vi "设备-初始化配置.vi"() -> ()   [LabVIEW 2013]
uses:
  <vilib>/Instr/_visa.llb/VISA Configure Serial Port (Instr).vi
panel:
  out "配置服务器VI引用":refnum<vi>
  out "账户信息":string caption="* 提示："
  out "服务器？":bool
  out "路由？":bool
  out "通信？":bool
  in  "刷新服务器":bool
  in  "连接的设备":i32(listbox)
  in  "配置开关":bool
  out "配置进度":dbl(slide) scale=0.0..1.0
  out "本机IP":string
  out "IP":string
  out "端口":u16
  in  "当前配置流程":T1(ring)
  in  "连续配置":bool=TRUE
  out "MAC":string
  out "查MAC回复":string
  in  "路由密码":string caption="* 路由密码"
  out "路由名称":string
  in  "通信接口":refnum<visa-resource-name> caption="* 通信接口"
  # "已连接设备"
  # "与设备连接"
  # "设备连接到路由器"
  # "设备连接到服务器"
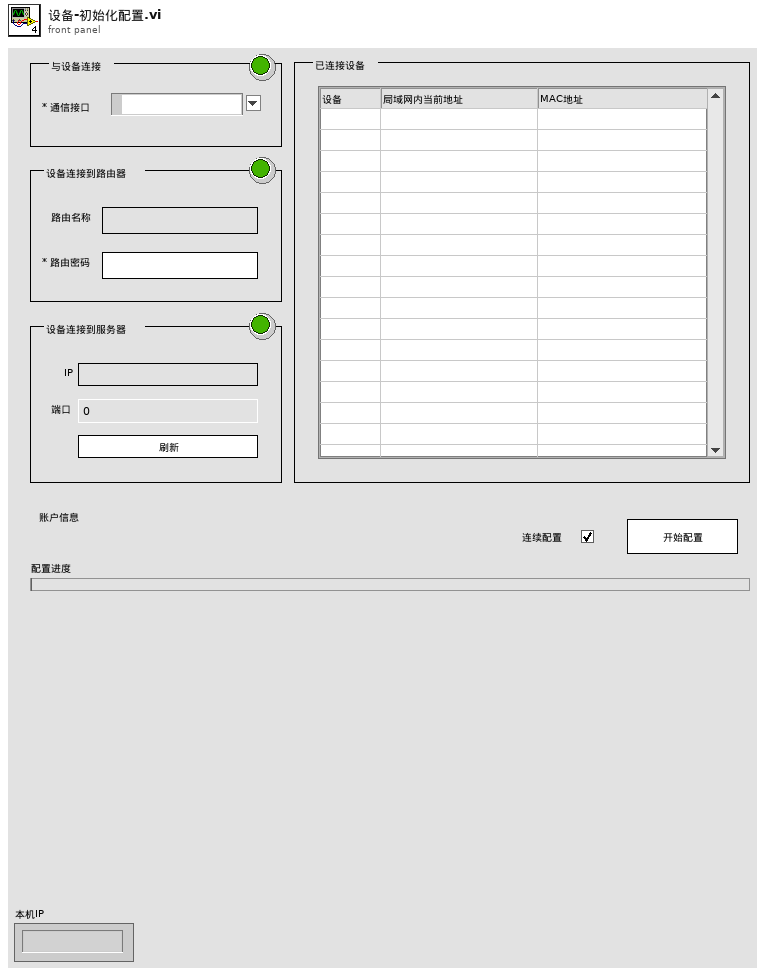
[diagram p1: front panel]
types:
  T1 = enum16{"退出透传", "进入AT指令", "退出AP连接", "设为STA", "连接指定AP", "设为STA开机自连", "获取MAC地址", "禁用智能连接", "透传接收", "连接至配置服务器", "进入透传发送", "等待云服务器端确认", "配置完成"}
  T2 = enum8{"Enabled", "Disabled", "Disabled and Grayed Out"}
  T3 = cluster{"服务器信息":cluster{"IP":string, "Port":u16}, "账户信息":cluster{"账户可用？":bool, "用户名":string, "密码":string}}
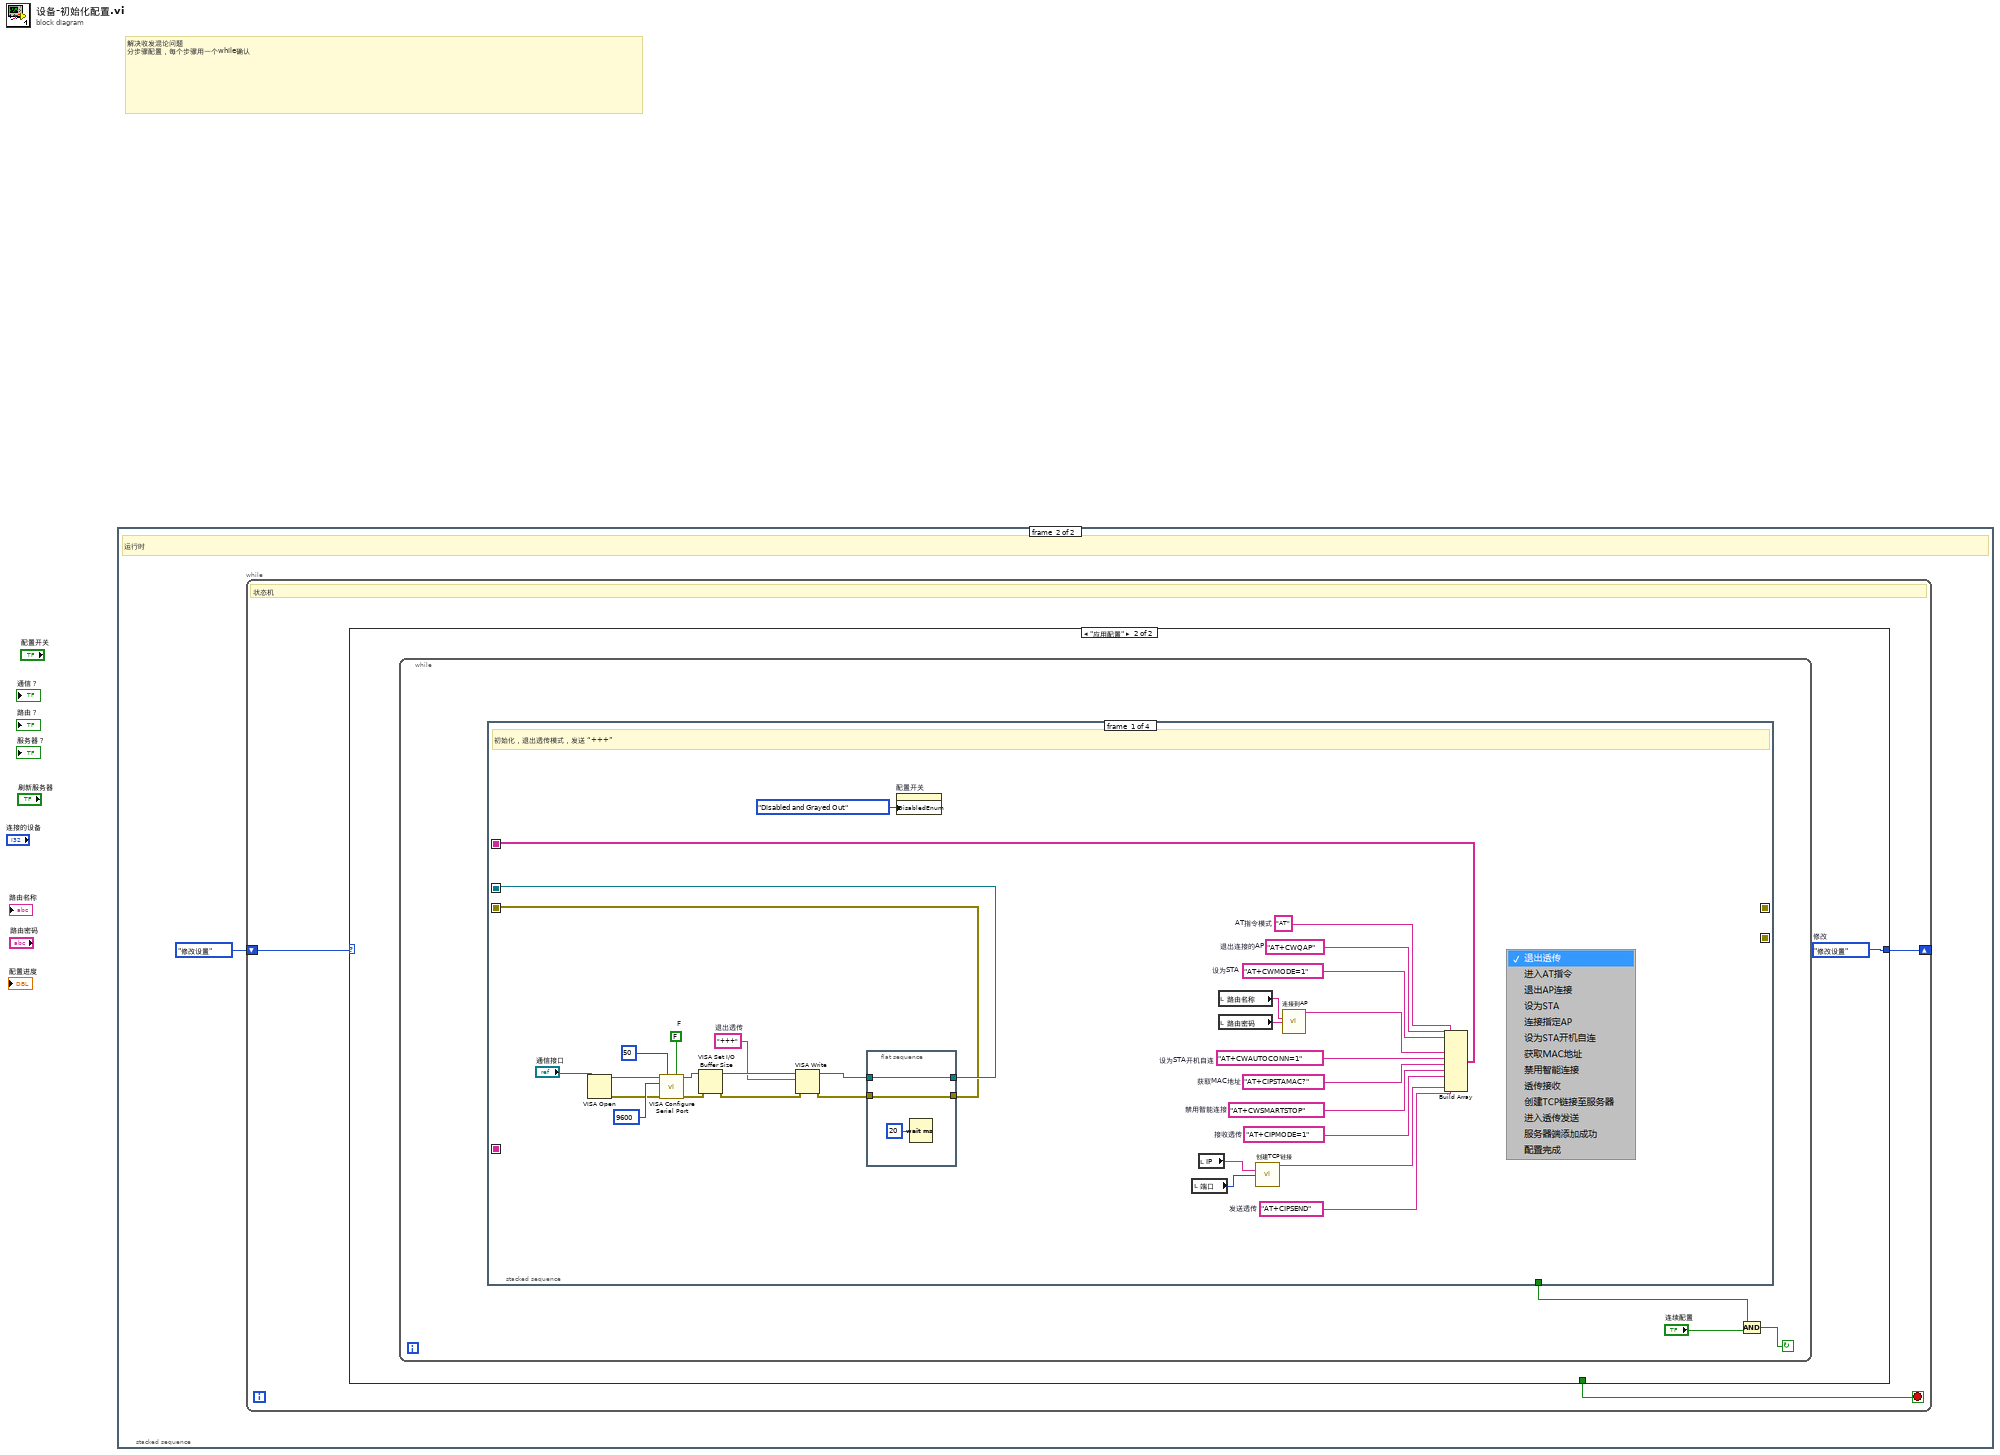
[diagram p0: block diagram]
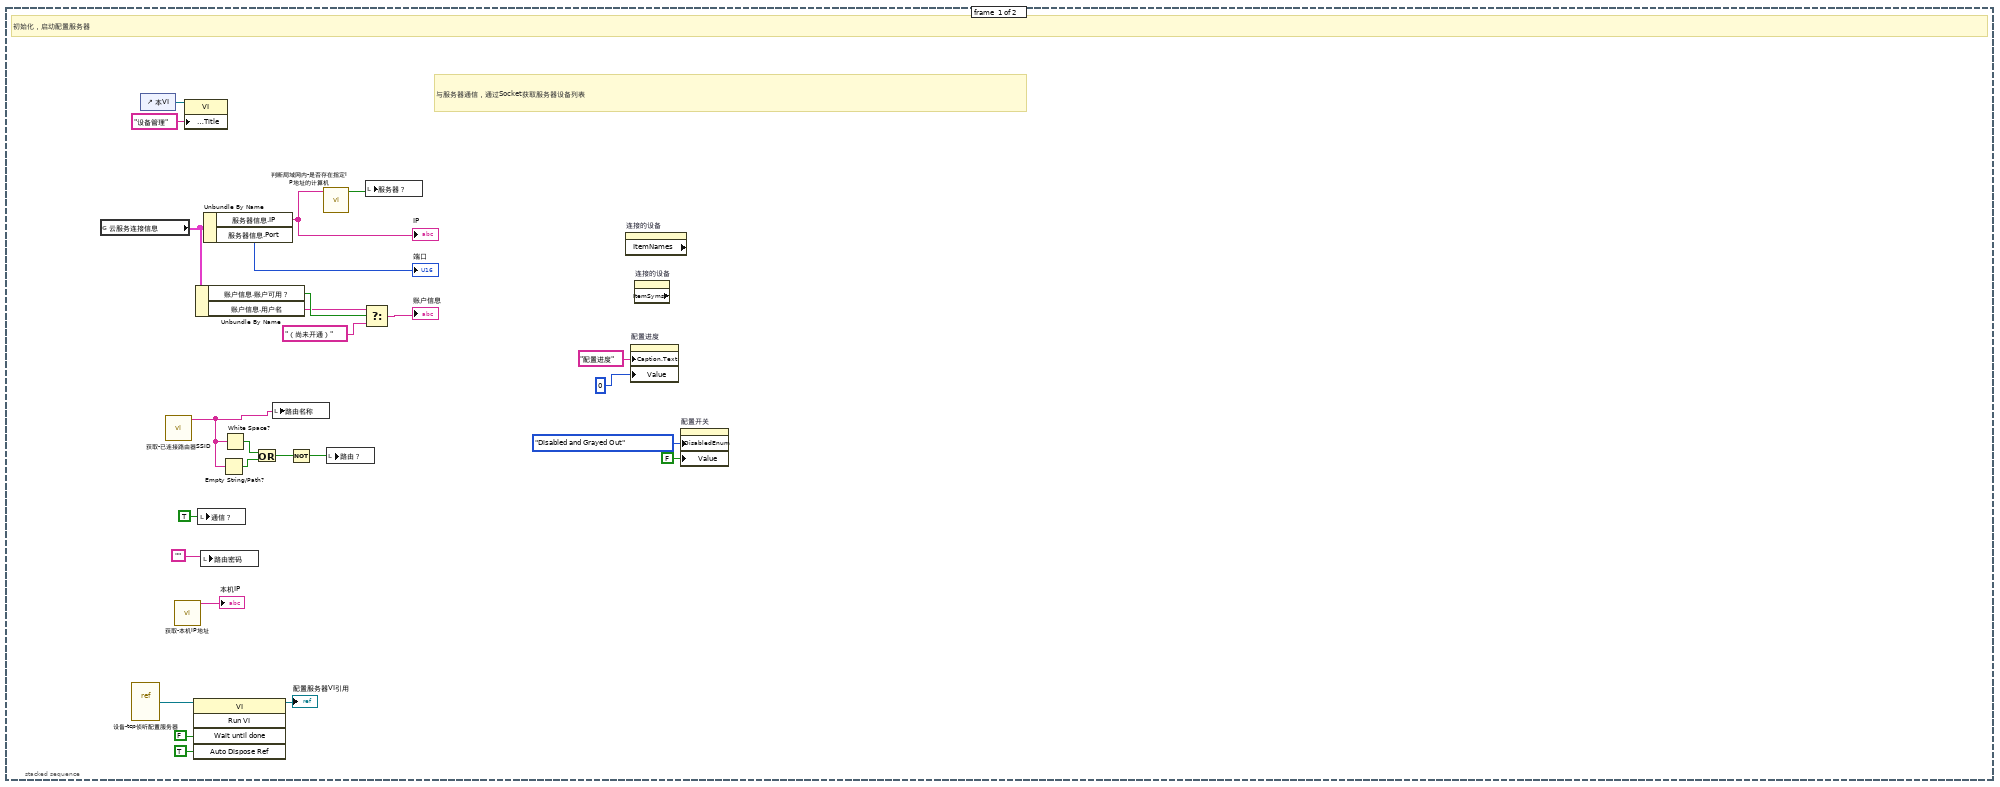
[diagram p2: hidden frame]
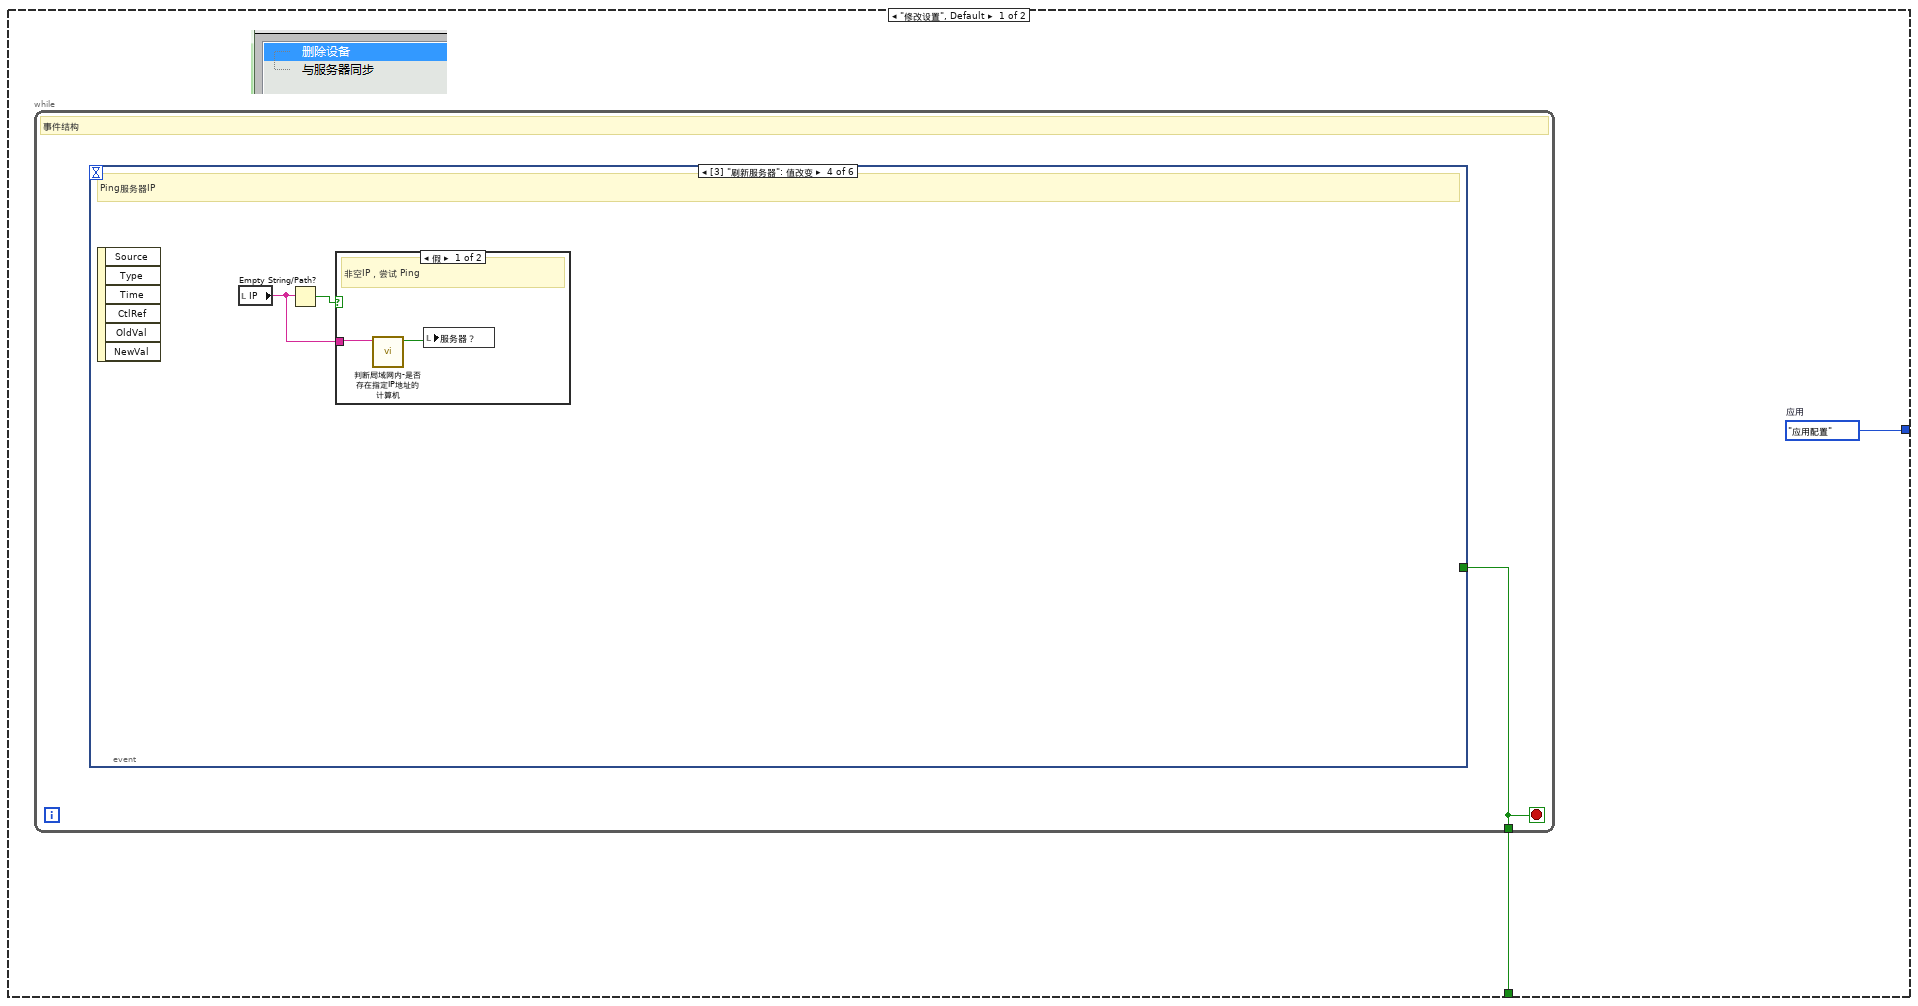
[diagram p3: hidden frame]
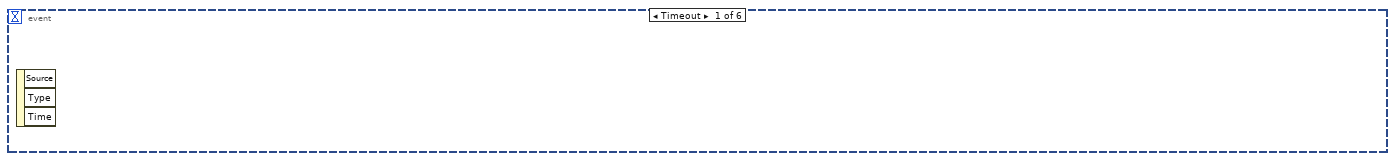
[diagram p4: hidden frame]
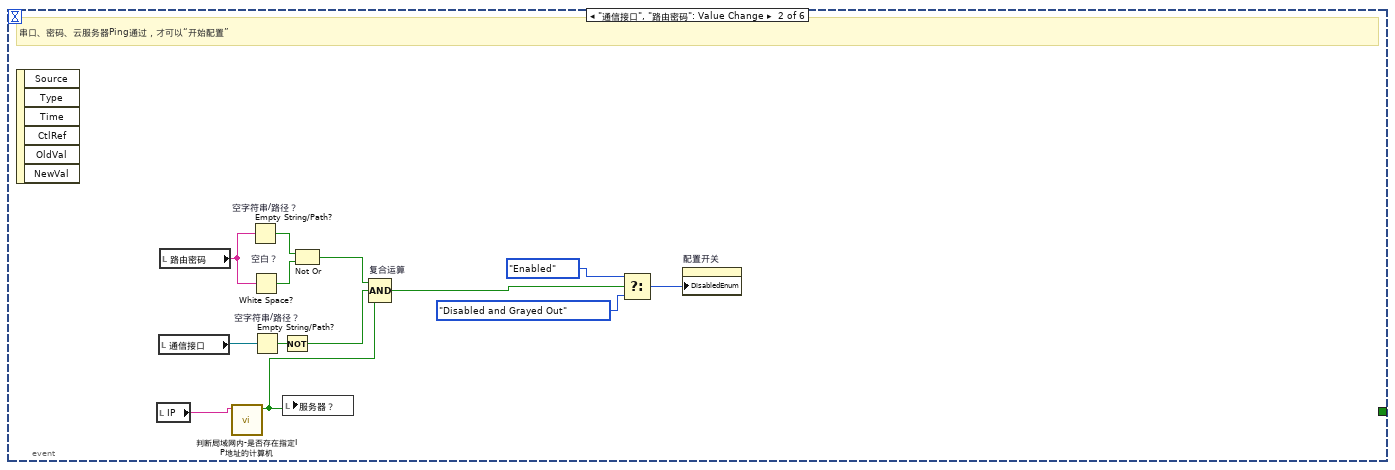
[diagram p5: hidden frame]
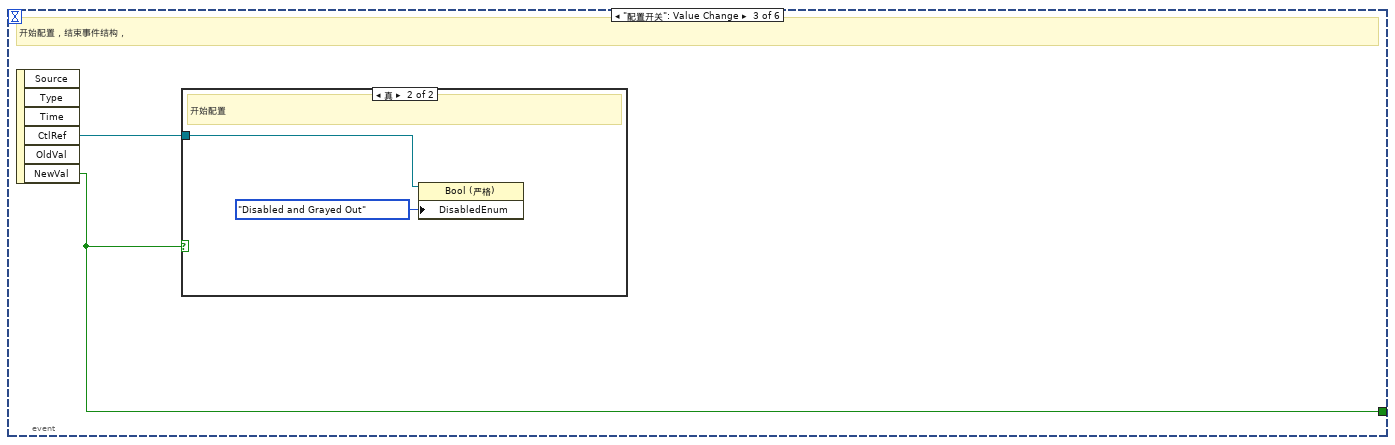
[diagram p6: hidden frame]
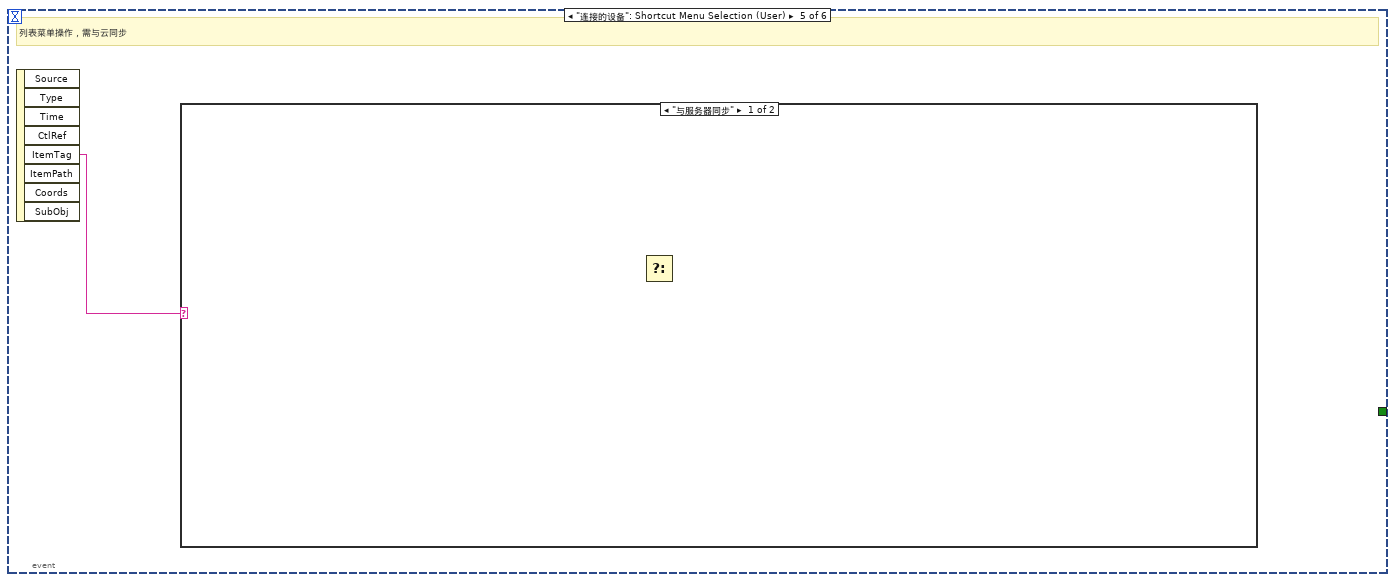
[diagram p9: hidden frame]
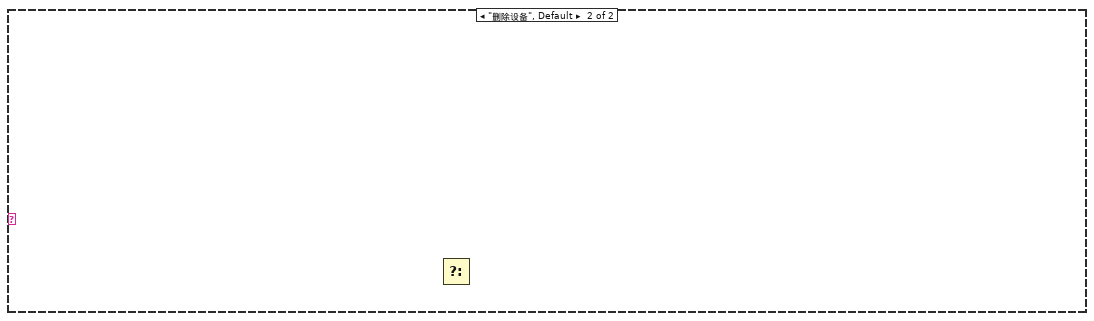
[diagram p10: hidden frame]
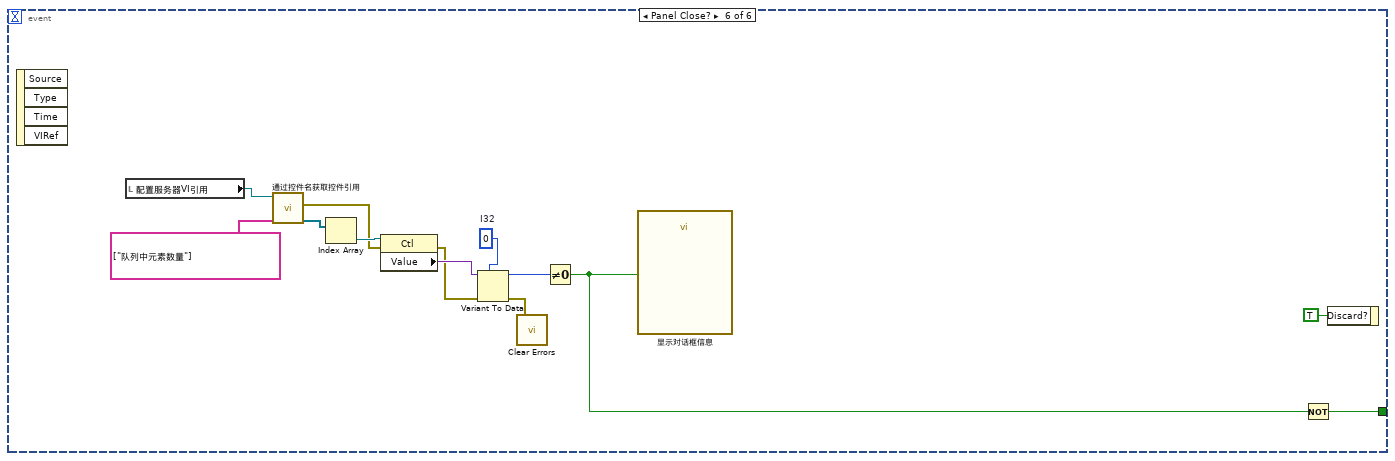
[diagram p11: hidden frame]
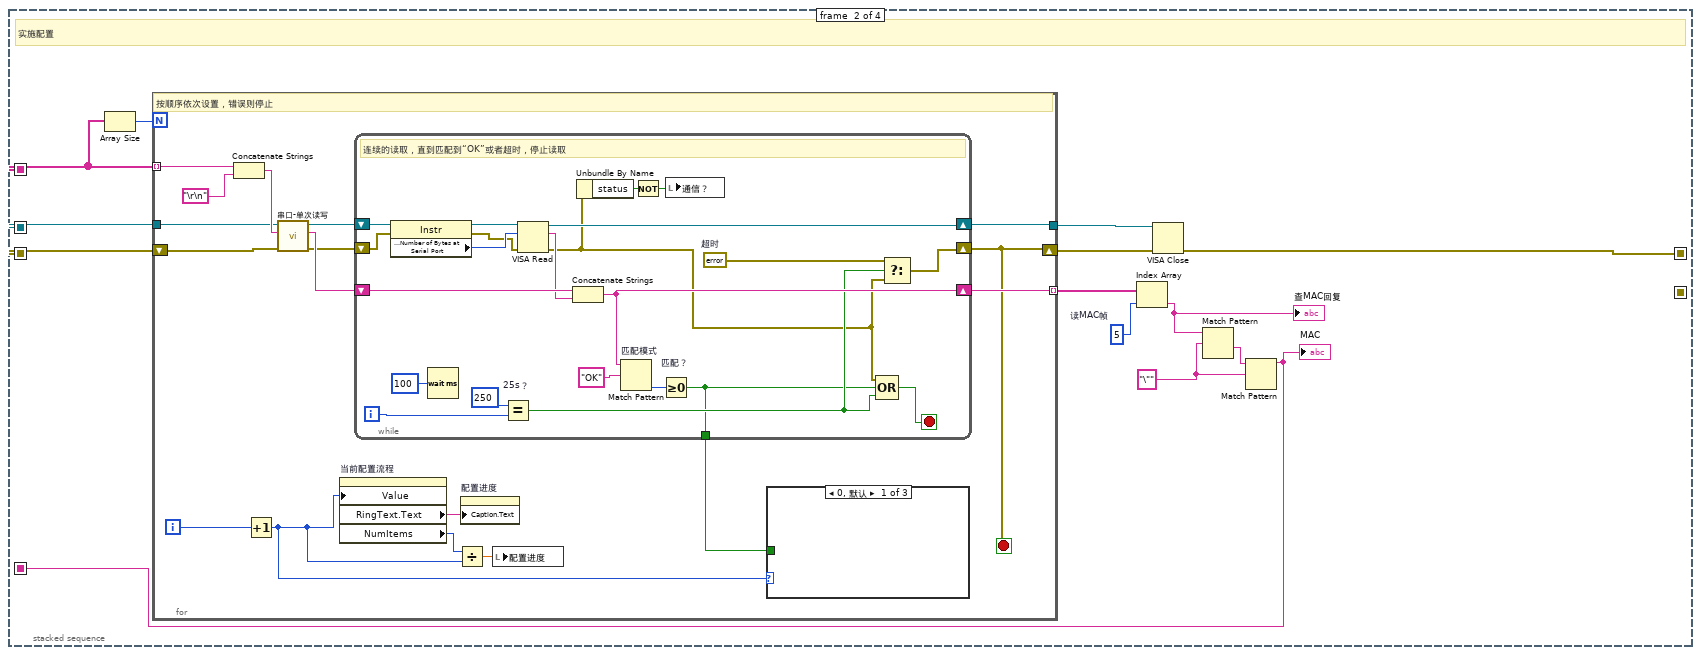
[diagram p12: hidden frame]
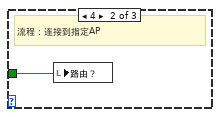
[diagram p13: hidden frame]
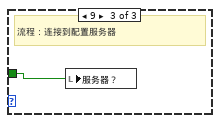
[diagram p14: hidden frame]
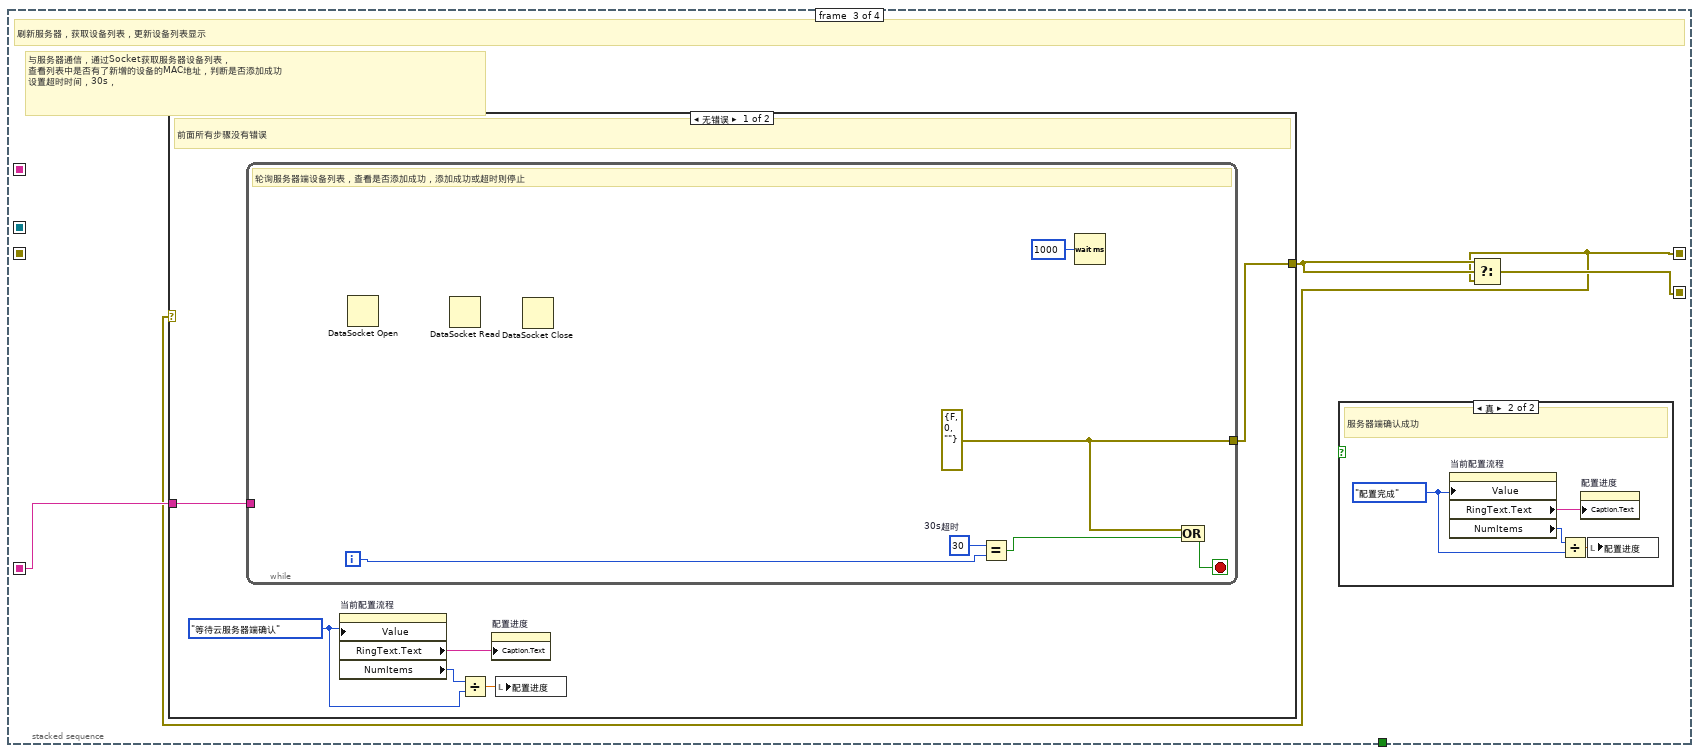
[diagram p15: hidden frame]
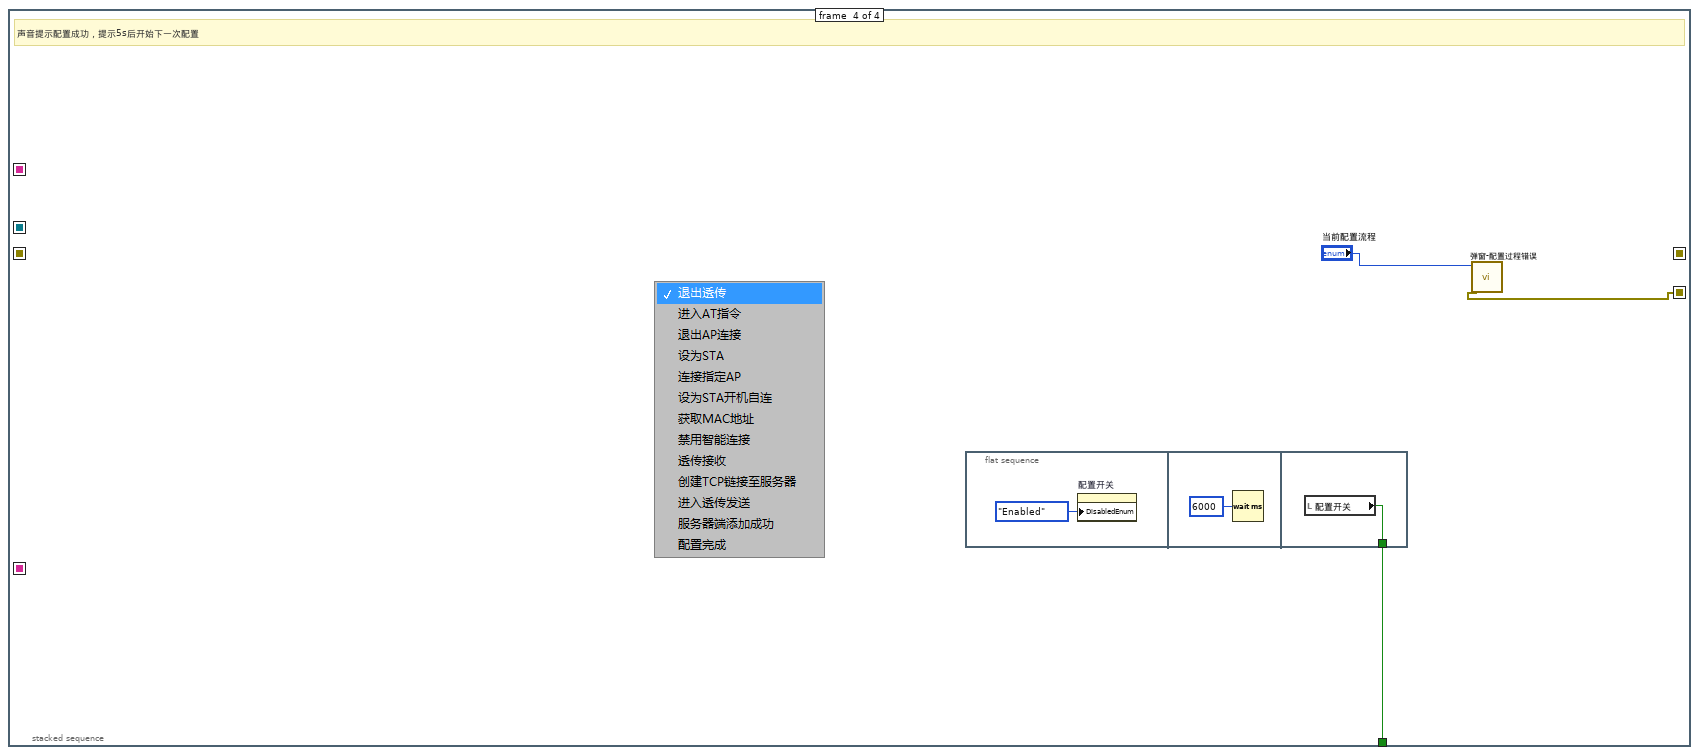
[diagram p18: hidden frame]
diagram:
  # "解决收发混论问题\n分步骤配置，每个步骤用一个while确认"
  n1 = stacked-sequence {
    frame #0 {
      # "与服务器通信，通过Socket获取服务器设备列表"
      # "初始化，启动配置服务器"
      n2 = global read "Client-全局变量.vi" "云服务连接信息"() -> (w13:T3)
      n3 = vi-ref "设备-tcp侦听配置服务器.vi"() -> (w2:refnum<vi>)
      n4 = control-ref of="本VI"() -> (w24:refnum<vi>)
      n5 = call "获取-已连接路由器SSID.vi"() -> ("SSID"=w16:string)  [unwired: 11 in]
      n6 = call "获取-本机IP地址.vi"() -> ("本机IP"=→"本机IP":string)  [unwired: 10 in, 1 out]
      n7 = property class="VI"(reference=w24, "Front Panel.Title"="设备管理" ("前面板窗口:标题")) -> ()  [unwired: 1 in, 2 out]
      n8 = invoke class="VI" method="Run VI"(reference=w2, "Wait until done"=FALSE ("结束前等待"), "Auto Dispose Ref"=TRUE ("自动销毁引用")) -> (reference out=→"配置服务器VI引用":refnum<vi>)  [unwired: 2 in, 4 out]
      n9 = Unbundle By Name(w13) -> ("账户信息.账户可用？"=w12:bool, "账户信息.用户名"=w10:string)
      n10 = local write "通信？"(TRUE ("通信？")) -> ()
      n11 = local write "路由密码"("") -> ()
      n12 = Unbundle By Name(w13) -> ("服务器信息.IP"=w22:string, "服务器信息.Port"=→"端口":u16)
      "IP" <- w22
      n13 = Empty String/Path?(string/path=w16) -> (empty?=w20:bool)
      n14 = White Space?(1:w16) -> (0:w19:bool)
      n15 = Or(x=w19, y=w20) -> (x .or. y?=w18:bool)
      n16 = local write "路由名称"(w16) -> ()
      n17 = Not(x=w18) -> (.not. x?=w17:bool)
      n18 = call "判断局域网内-是否存在指定IP地址的计算机.vi"("IP地址"=w22) -> ("IP可用？"=w23:bool)  [unwired: 10 in]
      n19 = local write "路由？"(w17) -> ()
      n20 = Select(t=w10, s=w12, f="（尚未开通）" ("前面板窗口:标题")) -> (s? t:f=→"账户信息":string)
      n21 = local write "服务器？"(w23) -> ()
      n22 = property on="连接的设备" class="MCListbox (严格)" props=["ItemNames"]() -> ()  [unwired: 2 in, 3 out]
      n23 = property on="配置进度" class="滑动杆 (严格)"("Caption.Text"="配置进度" ("标题.文本"), "Value"=u8 0 ("配置进度")) -> ()  [unwired: 2 in, 2 out]
      n24 = property on="连接的设备" class="多列列表框 (严格)" props=["ItemSyms"]() -> ()  [unwired: 2 in, 3 out]
      n25 = property on="配置开关" class="Bool (严格)"("DisabledEnum"=T2."Disabled and Grayed Out" ("禁用"), "Value"=FALSE ("配置开关")) -> ()  [unwired: 2 in, 2 out]
    }
    frame #1 {
      # "运行时"
      n26 = while {
        shift-right: [w28] -> _
        shift-left: enum16{"修改设置", "应用配置"}."修改设置" -> [w30]
        stop <- w29 stop-if-true
        # "状态机"
        n27 = case shown="\"应用配置\"" w30 {
          tunnel: [w32 _] -> w29
          tunnel: [w31 w69] -> w28
          frame "修改设置", Default {
            w31 = enum16{"修改设置", "应用配置"}."应用配置"  # 应用
            n28 = while {
              tunnel: [w33] -> w32
              stop <- w33 stop-if-true
              # "事件结构"
              n29 = event shown="[3] \"刷新服务器\": 值改变" {
                selector: _ -> [_ _ _ _ _ _]
                dyn-events: _ -> [_ _ _ _ _ _]
                timeout: _ -> [_ _ _ _ _ _]
                tunnel: [_ _ w47 _ _ w56] -> w33
                event Timeout {
                  n30 = event-data() -> ()  [unwired: 1 in, 3 out]
                }
                event "通信接口", "路由密码": Value Change {
                  # "串口、密码、云服务器Ping通过，才可以“开始配置”"
                  n31 = event-data() -> ()  [unwired: 1 in, 6 out]
                  n32 = local read "IP"() -> (w35:string)
                  n33 = local read "通信接口"() -> (w43:refnum<visa-resource-name>)
                  n34 = local read "路由密码"() -> (w46:string)
                  n35 = call "判断局域网内-是否存在指定IP地址的计算机.vi"("IP地址"=w35) -> ("IP可用？"=w34:bool)  [unwired: 10 in]
                  n36 = Empty String/Path? "空字符串/路径？"(string/path=w46) -> (empty?=w44:bool)
                  n37 = White Space? "空白？"(1:w46) -> (0:w45:bool)
                  n38 = Empty String/Path? "空字符串/路径？"(string/path=w43) -> (empty?=w42:bool)
                  n39 = Not(x=w42) -> (.not. x?=w40:bool)
                  n40 = local write "服务器？"(w34) -> ()
                  n41 = Not Or(1:w45, 2:w44) -> (0:w41:bool)
                  n42 = Compound Arithmetic op=AND "复合运算"(w41, w40, w34) -> (w39:bool)
                  n43 = Select(t=T2."Enabled" ("禁用"), s=w39, f=T2."Disabled and Grayed Out" ("禁用")) -> (s? t:f=w36:T2)
                  n44 = property on="配置开关" class="Bool (严格)"("DisabledEnum"=w36) -> ()  [unwired: 2 in, 2 out]
                }
                event "配置开关": Value Change {
                  # "开始配置，结束事件结构，"
                  n45 = event-data() -> ("CtlRef"=w48:refnum<vi>, "NewVal"=w47:bool)  [unwired: 1 in, 4 out]
                  n46 = case shown="真" w47 {
                    tunnel: w48 -> [_ w49]
                    frame False {
                    }
                    frame True {
                      # "开始配置"
                      n47 = property class="Bool (严格)"(reference=w49, "DisabledEnum"=T2."Disabled and Grayed Out" ("禁用")) -> ()  [unwired: 1 in, 2 out]
                    }
                  }
                }
                event "刷新服务器": Value Change {
                  # "Ping服务器IP"
                  n48 = event-data() -> ()  [unwired: 1 in, 6 out]
                  n49 = local read "IP"() -> (w51:string)
                  n50 = Empty String/Path?(string/path=w51) -> (empty?=w52:bool)
                  n51 = case shown="假" w52 {
                    tunnel: w51 -> [w53 _]
                    frame False {
                      # "非空IP，尝试 Ping"
                      n52 = call "判断局域网内-是否存在指定IP地址的计算机.vi"("IP地址"=w53) -> ("IP可用？"=w54:bool)  [unwired: 10 in]
                      n53 = local write "服务器？"(w54) -> ()
                    }
                    frame True {
                      # "空IP地址，不执行"
                    }
                  }
                }
                event "连接的设备": Shortcut Menu Selection (User) {
                  # "列表菜单操作，需与云同步"
                  n54 = event-data() -> ("ItemTag"=w55:string)  [unwired: 1 in, 7 out]
                  n55 = case shown="\"与服务器同步\"" w55 {
                    frame "与服务器同步" {
                      n56 = Select() -> ()  [unwired: 3 in, 1 out]
                    }
                    frame "删除设备", Default {
                      n57 = Select() -> ()  [unwired: 3 in, 1 out]
                    }
                  }
                }
                event Panel Close? {
                  w63 = 0  # I32
                  n58 = event-data() -> ()  [unwired: 1 in, 4 out]
                  n59 = local read "配置服务器VI引用"() -> (w68:refnum<vi>)
                  n60 = call "通过控件名获取控件引用.vi"("控件名数组"=string[] ["队列中元素数量"], "VI引用"=w68) -> ("控件引用输出"=w66:refnum<vi>[], "错误输出"=w62:errorcluster)  [unwired: 7 in, 1 out]
                  n61 = Index Array(array=w66) -> (element=w65:refnum<vi>)  [unwired: 1 in]
                  n62 = property class="Ctl"(reference=w65, error in=w62) -> (error out=w61:errorcluster, "Value"=w64:variant)  [unwired: 1 out]
                  n63 = Variant To Data(error in=w61, type=w63, Variant=w64) -> (data=w59:i32, error out=w60:errorcluster)
                  n64 = call <vilib>:"Clear Errors.vi"("error in (no error)"=w60) -> ()  [unwired: 6 in, 1 out]
                  n65 = Not Equal To 0?(x=w59) -> (x != 0?=w57:bool)
                  n66 = call "显示对话框信息"("Enable"=w57) -> ()  [unwired: 9 in, 2 out]
                  n67 = Not(x=w57) -> (.not. x?=w56:bool)
                  n68 = event-data("Discard?"=TRUE ("放弃？")) -> ()  [unwired: 1 in, 1 out]
                }
              }
            }
          }
          frame "应用配置" {
            w69 = enum16{"修改设置", "应用配置"}."修改设置"  # 修改
            n69 = while {
              stop <- w72 continue-if-true
              n70 = stacked-sequence {
                seq-local: [w90 _ _ _] -> [_ w119 _ _]
                seq-local: [w89 _ _ _] -> [_ w118 _ _]
                seq-local: [_ w110 _ _] -> [_ _ w161 _]
                seq-local: [w74 _ _ _] -> [_ w109 _ _]
                seq-local: [_ w108 _ _] -> [_ _ w164 _]
                seq-local: [_ _ w162 _] -> [_ _ _ w183]
                tunnel: [_ _ _ w182] -> w70
                frame #0 {
                  w88 = "AT+CIPSEND"  # 发送透传
                  w86 = "AT+CIPMODE=1"  # 接收透传
                  w85 = "AT+CWSMARTSTOP"  # 禁用智能连接
                  w84 = "AT+CIPSTAMAC?"  # 获取MAC地址
                  w83 = "AT+CWAUTOCONN=1"  # 设为STA开机自连
                  w81 = "AT+CWMODE=1"  # 设为STA
                  w80 = "AT+CWQAP"  # 退出连接的AP
                  w79 = "AT"  # AT指令模式
                  w95 = "+++"  # 退出透传
                  w98 = FALSE  # F
                  # "初始化，退出透传模式，发送 “+++”"
                  n71 = VISA Open(VISA resource name="通信接口") -> (VISA resource name=w100:refnum<visa-resource-name>, error out=w99:errorcluster)  [unwired: 1 in, 3 out]
                  n72 = call-poly "VISA Configure Serial Port"("VISA resource name"=w100, "timeout (10sec)"=u32 50, "Enable Termination\nChar (T)"=w98, "baud rate (9600)"=u32 9600, "error in (no error)"=w99) -> ("VISA resource name out"=w103:refnum<visa-resource-name>, "error out"=w93:errorcluster)  [unwired: 3 in, 6 out]
                  n73 = VISA Set I/O Buffer Size(VISA resource name=w103, error in (no error)=w93) -> (VISA resource name out=w96:refnum<visa-resource-name>, error out=w94:errorcluster)  [unwired: 2 in]
                  n74 = VISA Write(VISA resource name=w96, write buffer=w95, error in (no error)=w94) -> (VISA resource name out=w92:refnum<visa-resource-name>, error out=w91:errorcluster)  [unwired: 1 out]
                  n75 = flat-sequence {
                    tunnel: w92 -> [w105]
                    tunnel: w91 -> [w104]
                    tunnel: [w105] -> w90
                    tunnel: [w104] -> w89
                    frame #0 {
                      n76 = Wait (ms)(milliseconds to wait=u32 20 ("等待时间（毫秒）")) -> ()  [unwired: 1 out]
                    }
                  }
                  n77 = property on="配置开关" class="Bool (严格)"("DisabledEnum"=T2."Disabled and Grayed Out" ("禁用")) -> ()  [unwired: 2 in, 2 out]
                  n78 = local read "端口"() -> (w75:u16)
                  n79 = local read "IP"() -> (w76:string)
                  n80 = local read "路由名称"() -> (w78:string)
                  n81 = local read "路由密码"() -> (w77:string)
                  n82 = call "创建TCP链接"("服务器IP"=w76, "服务器Port"=w75) -> ("Result"=w87:string)  [unwired: 12 in, 1 out]
                  n83 = call "连接到AP"("路由名称"=w78, "路由密码"=w77) -> ("Result"=w82:string)  [unwired: 12 in, 1 out]
                  n84 = Build Array(w79, w80, w81, w82, w83, w84, w85, w86, w87, w88) -> (w74:string[])
                }
                frame #1 {
                  w115 = "\"" ("搜索字符串/字符(-)")
                  w116 = 5  # 读MAC帧
                  # "实施配置"
                  n85 = Array Size(array=w109) -> (size(s)=w107:i32)
                  n86 = for {
                    N: w107 -> [_]
                    tunnel: w109 -> [w136] mode=indexing
                    tunnel: w119 -> [w134]
                    shift-right: [w127] -> w111
                    shift-left: w118 -> [w133]
                    tunnel: [w128] -> w117 mode=indexing
                    tunnel: [w126] -> w112
                    i -> [w125]
                    stop <- w127 stop-if-true
                    # "按顺序依次设置，错误则停止"
                    n87 = Concatenate Strings(w136, "\r\n") -> (w135:string)
                    n88 = Increment(x=w125) -> (x+1=w121:i32)
                    n89 = call "串口-单次读写.vi"("错误输入（无错误）"=w133, "写入缓冲区"=w135, "VISA资源名称"=w134) -> ("错误输出"=w129:errorcluster, "读取缓冲区"=w131:string, "VISA资源名称输出"=w130:refnum<visa-resource-name>)  [unwired: 6 in]
                    n90 = property on="当前配置流程" class="枚举 (严格)"("Value"=w121) -> ("RingText.Text"=w123:string, "NumItems"=w122:u32)  [unwired: 2 in, 2 out]
                    n91 = while {
                      shift-right: [w150] -> w128
                      shift-left: w131 -> [w152]
                      shift-right: [w155] -> w126
                      shift-left: w130 -> [w156]
                      shift-right: [w143] -> w127
                      shift-left: w129 -> [w154]
                      tunnel: [w139] -> w120
                      i -> [w148]
                      stop <- w146 stop-if-true
                      w144 = errorcluster {"status"=TRUE, "code"=0, "source"="等不及了"}  # 超时
                      # "连续的读取，直到匹配到“OK”或者超时，停止读取"
                      n92 = property class="Instr"(reference=w156, error in=w154) -> (reference out=w160:refnum<visa-resource-name>, error out=w153:errorcluster, "Serial Settings:Number of Bytes at Serial Port"=w159:u32)
                      n93 = Wait (ms)(milliseconds to wait=u32 100 ("等待时间（毫秒）")) -> ()  [unwired: 1 out]
                      n94 = Equal? "25s？"(x=250, y=w148) -> (x = y?=w145:bool)
                      n95 = VISA Read(VISA resource name=w160, byte count=w159, error in (no error)=w153) -> (VISA resource name out=w155:refnum<visa-resource-name>, read buffer=w151:string, error out=w142:errorcluster)  [unwired: 1 out]
                      n96 = Concatenate Strings(w152, w151) -> (w150:string)
                      n97 = Unbundle By Name(w142) -> ("status"=w141:bool)
                      n98 = Match Pattern "匹配模式"(string=w150, regular expression="OK" ("正则表达式")) -> (offset past match=w158:i32)  [unwired: 1 in, 3 out]
                      n99 = Not(x=w141) -> (.not. x?=w140:bool)
                      n100 = Greater Or Equal To 0? "匹配？"(x=w158) -> (x >= 0?=w139:bool)
                      n101 = local write "通信？"(w140) -> ()
                      n102 = Compound Arithmetic op=OR ("复合运算")(w142, w139, w145) -> (w146:bool)
                      n103 = Select(t=w144, s=w145, f=w142) -> (s? t:f=w143:errorcluster)
                    }
                    n104 = Divide(x=w122, y=w121) -> (x/y=w124:dbl)
                    n105 = property on="配置进度" class="滑动杆 (严格)"("Caption.Text"=w123) -> ()  [unwired: 2 in, 2 out]
                    n106 = local write "配置进度"(w124) -> ()
                    n107 = case shown="0, 默认" w121 {
                      tunnel: w120 -> [_ w137 w138]
                      frame 0, Default {
                      }
                      frame 4 {
                        # "流程：连接到指定AP"
                        n108 = local write "路由？"(w137) -> ()
                      }
                      frame 9 {
                        # "流程：连接到配置服务器"
                        n109 = local write "服务器？"(w138) -> ()
                      }
                    }
                  }
                  n110 = Index Array(array=w117, index=w116) -> (element=w114:string)
                  "查MAC回复" <- w114
                  n111 = VISA Close(VISA resource name=w112, error in (no error)=w111) -> (error out=w110:errorcluster)
                  n112 = Match Pattern(string=w114, regular expression=w115) -> (after substring=w113:string)  [unwired: 1 in, 3 out]
                  n113 = Match Pattern(string=w113, regular expression=w115) -> (before substring=w108:string)  [unwired: 1 in, 3 out]
                  "MAC" <- w108
                }
                frame #2 {
                  # "与服务器通信，通过Socket获取服务器设备列表，\n查看列表中是否有了新增的设备的MAC地址，判断是否添加成功\n设置超时时间，30s，"
                  # "刷新服务器，获取设备列表，更新设备列表显示"
                  n114 = case shown="无错误" w161 {
                    selector: w161 -> [_ w177]
                    tunnel: w164 -> [w170 _]
                    tunnel: [w169 w177] -> w163
                    frame No Error {
                      w165 = T1."等待云服务器端确认" ("当前配置流程")
                      # "前面所有步骤没有错误"
                      n115 = while {
                        tunnel: w170 -> [_]
                        tunnel: [w171] -> w169
                        i -> [w175]
                        stop <- w172 stop-if-true
                        w171 = errorcluster {"status"=FALSE, "code"=0, "source"=""} ("错误输出")
                        w174 = 30  # 30s超时
                        # "轮询服务器端设备列表，查看是否添加成功，添加成功或超时则停止"
                        n116 = DataSocket Open() -> ()  [unwired: 4 in, 2 out]
                        n117 = DataSocket Read() -> ()  [unwired: 5 in, 7 out]
                        n118 = DataSocket Close() -> ()  [unwired: 3 in, 2 out]
                        n119 = Equal?(x=w174, y=w175) -> (x = y?=w173:bool)
                        n120 = Wait (ms)(milliseconds to wait=u32 1000 ("等待时间（毫秒）")) -> ()  [unwired: 1 out]
                        n121 = Compound Arithmetic op=OR(w171, w173) -> (w172:bool)
                      }
                      n122 = property on="当前配置流程" class="枚举 (严格)"("Value"=w165) -> ("RingText.Text"=w167:string, "NumItems"=w166:u32)  [unwired: 2 in, 2 out]
                      n123 = Divide(x=w166, y=w165) -> (x/y=w168:dbl)
                      n124 = property on="配置进度" class="滑动杆 (严格)"("Caption.Text"=w167) -> ()  [unwired: 2 in, 2 out]
                      n125 = local write "配置进度"(w168) -> ()
                    }
                    frame Error {
                      # "前面有步骤出现错误"
                    }
                  }
                  n126 = case shown="真" {
                    selector: _ -> [_ _]
                    frame False {
                      # "服务器端未确认"
                    }
                    frame True {
                      w178 = T1."配置完成" ("当前配置流程")
                      # "服务器端确认成功"
                      n127 = property on="当前配置流程" class="枚举 (严格)"("Value"=w178) -> ("RingText.Text"=w180:string, "NumItems"=w179:u32)  [unwired: 2 in, 2 out]
                      n128 = Divide(x=w179, y=w178) -> (x/y=w181:dbl)
                      n129 = property on="配置进度" class="滑动杆 (严格)"("Caption.Text"=w180) -> ()  [unwired: 2 in, 2 out]
                      n130 = local write "配置进度"(w181) -> ()
                    }
                  }
                  n131 = Select(t=w163, s=w163, f=w161) -> (s? t:f=w162:errorcluster)
                }
                frame #3 {
                  # "声音提示配置成功，提示5s后开始下一次配置"
                  n132 = flat-sequence {
                    tunnel: [w187] -> w182
                    frame #0 {
                      n133 = property on="配置开关" class="Bool (严格)"("DisabledEnum"=T2."Enabled" ("禁用")) -> ()  [unwired: 2 in, 2 out]
                    }
                    frame #1 {
                      n134 = Wait (ms)(milliseconds to wait=u32 6000 ("等待时间（毫秒）")) -> ()  [unwired: 1 out]
                    }
                    frame #2 {
                      n135 = local read "配置开关"() -> (w187:bool)
                    }
                  }
                  n136 = call "弹窗-配置过程错误.vi"("error int"=w183, "当前配置流程"="当前配置流程") -> ()  [unwired: 10 in]
                }
              }
              n137 = Compound Arithmetic op=AND(w70, "连续配置") -> (w72:bool)
            }
          }
        }
      }
    }
  }
